vi "Teardown.vi"(8 "Error in":errorcluster, 11 "Project Stuff in":refnum<class "Project Stuff.lvclass">) -> (0 "Error out":errorcluster)   [LabVIEW 2025, in "_Shared.lvlib" / "Project Stuff.lvclass"]
uses:
  Project Stuff.lvclass
  Project Stuff.lvclass/Project Stuff.ctl
  <vilib>/Utility/EditLVProj/Edit LVProj.lvlib
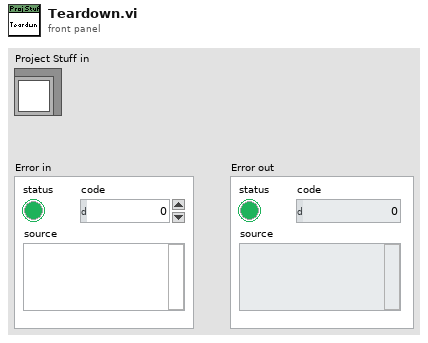
[diagram p1: front panel]
types:
  T1 = typedef "Edit LVProj.lvlib/Library And VI References.ctl" = cluster{"Target Reference":refnum<vi>, "VI References":refnum<vi>[], "Library References":refnum<vi>[]}
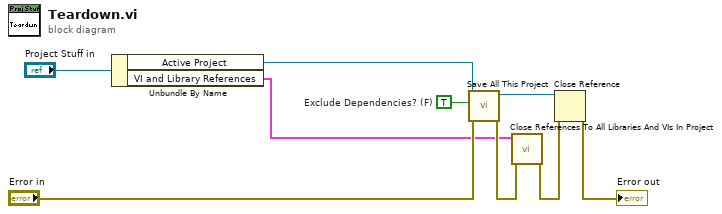
[diagram p0: block diagram]
diagram:
  w6 = TRUE  # Exclude Dependencies? (F)
  n1 = Unbundle By Name("Project Stuff in") -> ("Active Project"=w2:refnum<vi>, "VI and Library References"=w1:T1[])
  n2 = call <vilib>:"Save All This Project.vi"("error in (no error)"="Error in", "Exclude Dependencies? (F)"=w6, "Project in"=w2) -> ("error out"=w8:errorcluster, "Project out"=w7:refnum<vi>)  [unwired: 7 in]
  n3 = call <vilib>:"Close References To All Libraries And VIs In Project.vi"("error in (no error)"=w8, "VI and Library References"=w1) -> ("error out"=w9:errorcluster)  [unwired: 9 in]
  n4 = Close Reference(reference=w7, error in (no error)=w9) -> (error out=→"Error out":errorcluster)
